vi "Parse Input String.vi"(8 "error in (no error)":errorcluster, 10 "String":string, 11 "Alpaca Parser in":refnum<class "Parser.lvclass">) -> (0 "error out":errorcluster, 3 "Alpaca Parser out":refnum<class "Parser.lvclass">)   [LabVIEW 2019, in "JKI JSON Serialization.lvlib" / "Parser.lvclass"]
doc: "JKI JSON 1.1.10.37\nTomi Maila - JKI\nCopyright (c) 2017, JKI"
uses:
  Parser.lvclass
  Parser.lvclass/Parser.ctl
  Lexer/Lexer.lvclass
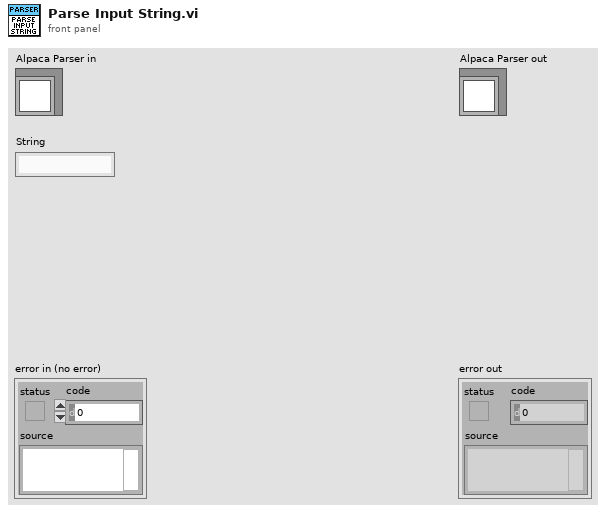
[diagram p1: front panel]
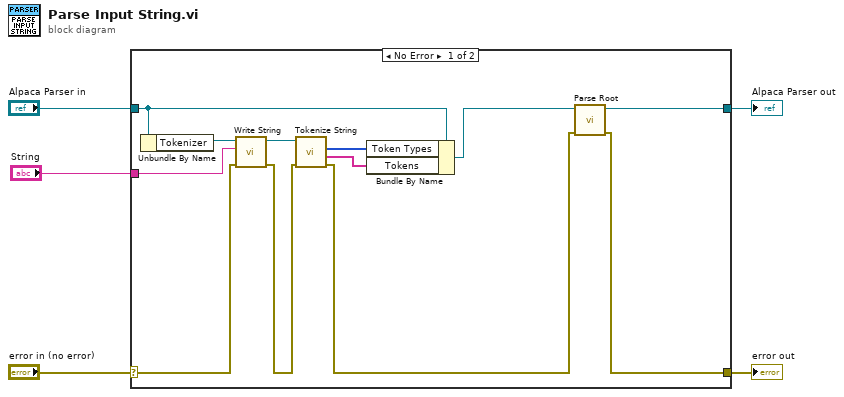
[diagram p0: block diagram]
diagram:
  n1 = case shown="No Error" "error in (no error)" {
    selector: "error in (no error)" -> [w15 w19]
    tunnel: [w6 w19] -> w4
    tunnel: [w8 w18] -> w2
    tunnel: "Alpaca Parser in" -> [w12 w18]
    tunnel: "String" -> [w16 _]
    frame No Error {
      n2 = Unbundle By Name(w12) -> ("Tokenizer"=w17:refnum<class "Lexer.lvclass">)
      n3 = call-dynamic "Write String.vi"("error in (no error)"=w15, "String"=w16, "Alpaca Tokenizer in"=w17) -> ("error out"=w13:errorcluster, "Alpaca Tokenizer out"=w14:refnum<class "Lexer.lvclass">)  [unwired: 7 in]
      n4 = call-dynamic "Tokenize String.vi"("error in (no error)"=w13, "Alpaca Tokenizer in"=w14) -> ("error out"=w7:errorcluster, "Tokens"=w10:string[], "Token Indices"=w11:i32[])  [unwired: 6 in, 1 out]
      n5 = Bundle By Name(cluster=w12, "Token Types"=w11, "Tokens"=w10) -> (w9:refnum<class "Parser.lvclass">)
      n6 = call-dynamic "Parse Root.vi"("error in (no error)"=w7, "Alpaca Parser in"=w9) -> ("error out"=w6:errorcluster, "Alpaca Parser out"=w8:refnum<class "Parser.lvclass">)  [unwired: 8 in]
    }
    frame Error {
    }
  }
  "error out" <- w4
  "Alpaca Parser out" <- w2
